vi "Execute Copy String Text.vi"(6 "Mouse Position":T1, 8 "User VI Ref":refnum<vi>, 9 "Menu Item Tag Suffix":string, 10 "Remaining Items":refnum<vi>[](array[refnum]), 11 "Affected Items":T2) -> (0 "Fail transaction?":bool)   [LabVIEW 2025]
doc: "This VI is part of a plug-in for modifying the LabVIEW shortcut menus. This is the execute VI which is called when the shortcut menu is chosen by the user. It performs the action of the selected menu item."
uses:
  Copy String Text.ctl
  <vilib>/Utility/miscctls.llb/LVPositionTypeDef.ctl
panel:
  out "error out":errorcluster
  # "All controls on this panel except \"Affected Items\" have been locked to prevent accidental edits. Changing the control names or types, other than the elements of the \"Affected Items\" cluster will make the VI unusable as a menu plugin.\n\nSee Context Help for each control for details about its use."
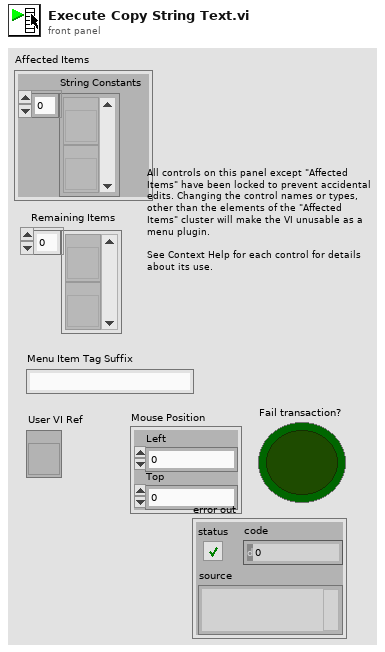
[diagram p1: front panel]
types:
  T1 = typedef "LVPositionTypeDef.ctl" = cluster{"Left":i32, "Top":i32}
  T2 = typedef "Copy String Text.ctl" = cluster{"String Constants":refnum<vi>[]}
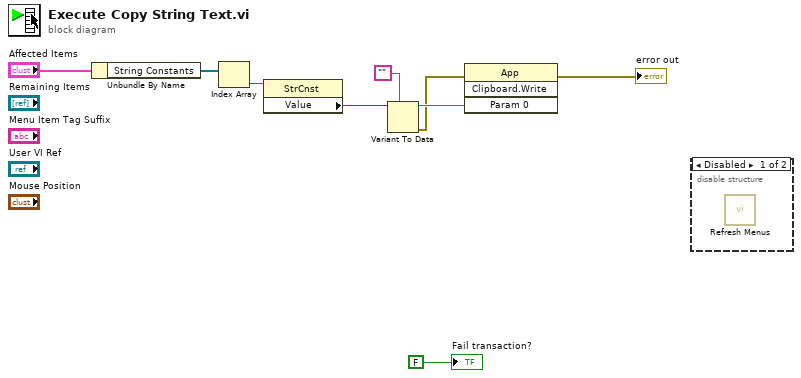
[diagram p0: block diagram]
diagram:
  n1 = Unbundle By Name("Affected Items") -> ("String Constants"=w7:refnum<vi>[])
  n2 = Index Array(array=w7) -> (element=w6:refnum<vi>)  [unwired: 1 in]
  n3 = property class="StrCnst"(reference=w6) -> ("Value"=w5:variant)  [unwired: 1 in, 2 out]
  n4 = Variant To Data(type="", Variant=w5) -> (data=w3:string, error out=w2:errorcluster)  [unwired: 1 in]
  n5 = invoke class="App" method="Clipboard.Write"(error in=w2, "Param 0"=w3) -> (error out=→"error out":errorcluster)  [unwired: 2 in, 3 out]
  n6 = disable-structure shown="Disabled" {
    frame Disabled {
      n7 = call <resource>:"Refresh Menus.vi"() -> ()  [unwired: 12 in]
    }
    frame Enabled {
    }
  }
  "Fail transaction?" <- FALSE ("Fail transaction?")
